vi "ZyklussteuerungGV-11-15.vi"(0 "Traps/MachKoeff0":dbl[](array[numeric]), 1 "DIOsNummern":cluster{"DIOsMod2BNr":i32[]}[](array[cluster]), 3 "FPGA VI Reference In":refnum<k20>, 5 "Traps/MachKoeff1":dbl[](array[numeric]), 7 "ServosWarmHigh (us)KaltHigh(us)":T1, 9 "Traps/MachKoeff2":dbl[](array[numeric]), 11 "Schieberegister":T2, 12 "Zeitpunkte/Setpoints":T4 {"FPGAPID"."proportional gain (Kc)" format="%.11g"; "FPGAPID"."integral gain (Kc*Ts/Ti)" format="%.11g"; "FPGAPID"."derivative gain (Kc*Td/Ts)" format="%.11g"}, 14 "MachKoeffs":T3) -> (4 "Schieberegister":T2)   [LabVIEW 2010]
uses:
  <vilib>/rvi/errors/niLvFpgaWhatHappensToTopLevelVI.ctl
  <vilib>/rvi/interface/common/niFpgaNodeNameForErrorReporting.ctl
  <vilib>/rvi/errors/niLvFpgaAdjustHostInterfaceError.vi
  <vilib>/rvi/interface/nirviReadWriteControl/nirviReadWriteControl.xnode
  GVZwangs.vi
  GVHorstSP.vi
  GVHeizenLH.vi
  GVVentilposition.vi
  GVZeitenZyklen.vi
  C:/Users/HAGAR-IV/Desktop/Zeugs/Johnny/pertrasgc fpga/FPGA-Programm-11-15.vi
  GVZwangsMPV.vi
  GVZwangsMPVPos.vi
  C:/Users/HAGAR-IV/Desktop/Zeugs/markus/version feb 2012/FPGA Bitfiles/pertrasgcfpga2_FPGATarget_FPGA-Programm-11_875D3646.lvbitx
  NiFpgaLv.dll
  <vilib>/Utility/error.llb/Error Cluster From Error Code.vi
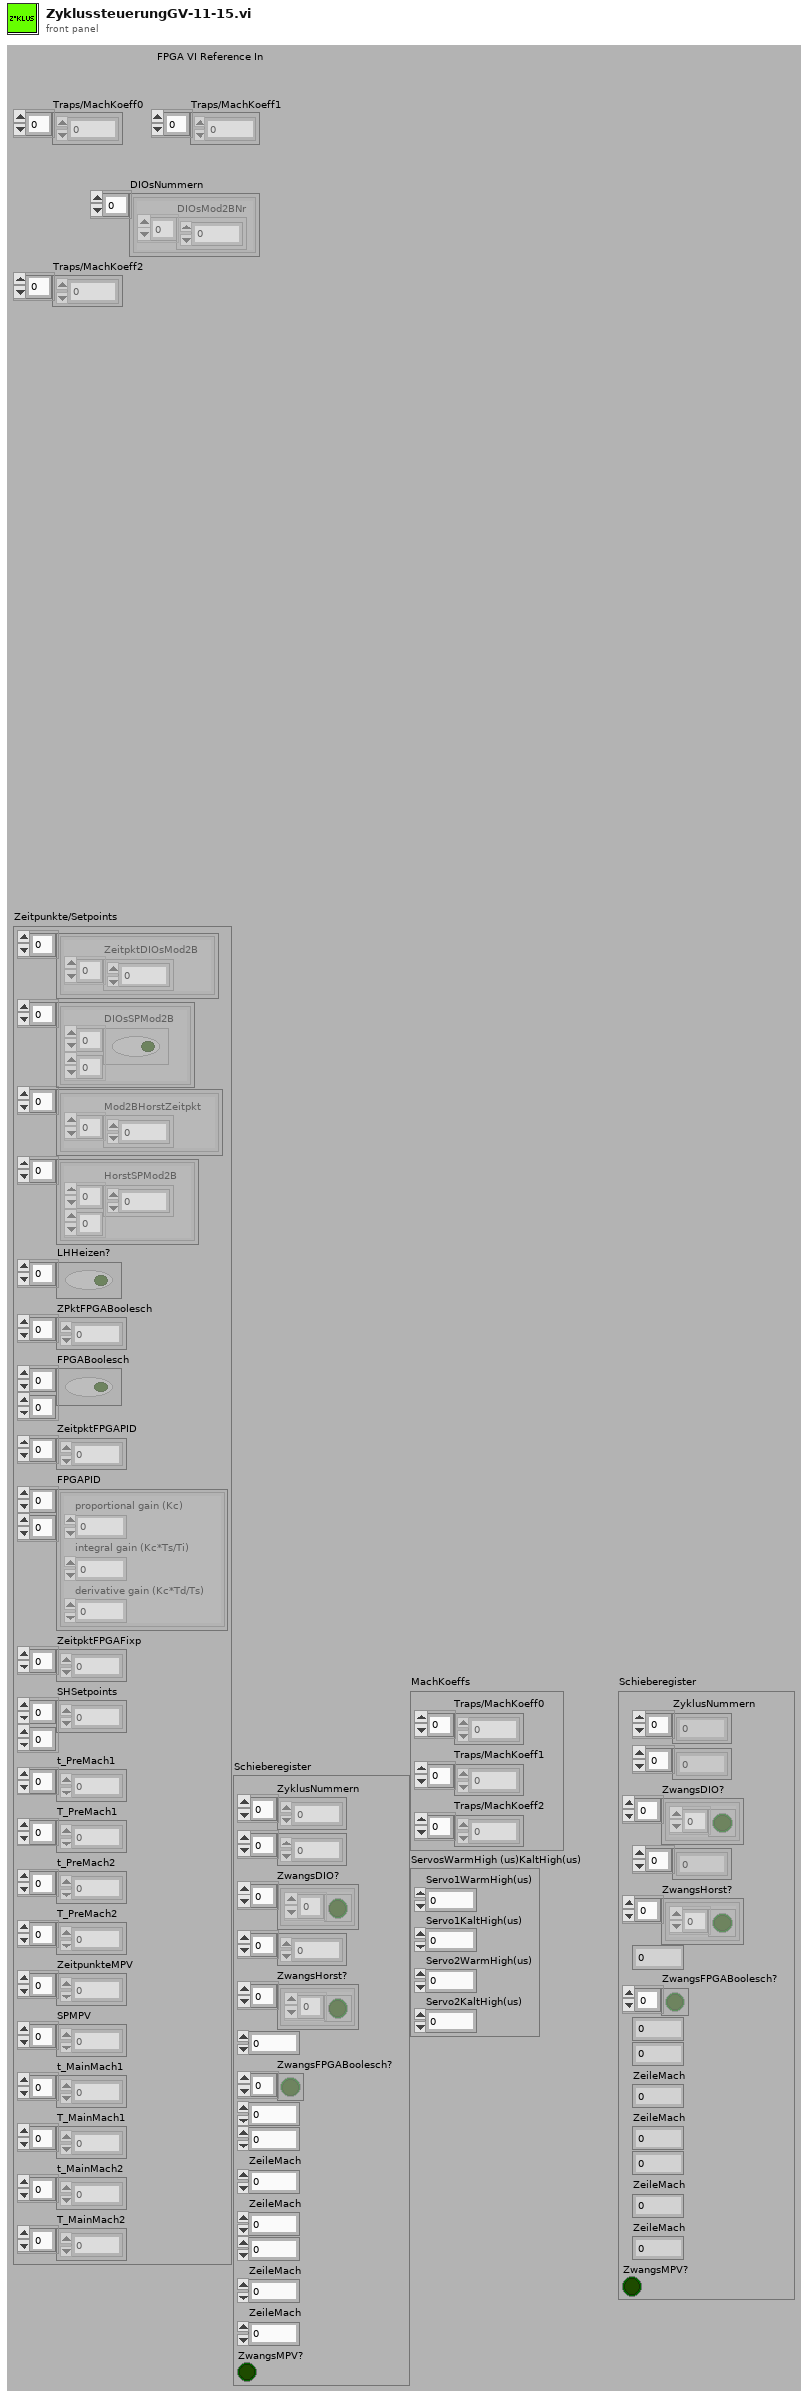
[diagram p1: front panel]
types:
  T1 = cluster{"Servo1WarmHigh(us)":u32, "Servo1KaltHigh(us)":u32, "Servo2WarmHigh(us)":u32, "Servo2KaltHigh(us)":u32}
  T2 = cluster{"ZyklusNummern":i32[], i32[], "ZwangsDIO?":cluster{bool[]}[], i32[], "ZwangsHorst?":cluster{bool[]}[], i32, "ZwangsFPGABoolesch?":bool[], i32, i32, "ZeileMach":i32, "ZeileMach":i32, i32, "ZeileMach":i32, "ZeileMach":i32, "ZwangsMPV?":bool}
  T3 = cluster{"Traps/MachKoeff0":dbl[], "Traps/MachKoeff1":dbl[], "Traps/MachKoeff2":dbl[]}
  T4 = cluster{cluster{"ZeitpktDIOsMod2B":dbl[]}[], cluster{"DIOsSPMod2B":bool[][]}[], cluster{"Mod2BHorstZeitpkt":dbl[]}[], cluster{"HorstSPMod2B":dbl[][]}[], "LHHeizen?":bool[], "ZPktFPGABoolesch":dbl[], "FPGABoolesch":bool[][], "ZeitpktFPGAPID":dbl[], "FPGAPID":cluster{"proportional gain (Kc)":fxp<+/-,16,8>, "integral gain (Kc*Ts/Ti)":fxp<+/-,16,8>, "derivative gain (Kc*Td/Ts)":fxp<+/-,16,8>}[][], "ZeitpktFPGAFixp":dbl[], "SHSetpoints":dbl[][], "t_PreMach1":dbl[], "T_PreMach1":dbl[], "t_PreMach2":dbl[], "T_PreMach2":dbl[], "ZeitpunkteMPV":dbl[], "SPMPV":i32[], "t_MainMach1":dbl[], "T_MainMach1":dbl[], "t_MainMach2":dbl[], "T_MainMach2":dbl[]}
  T5 = cluster{"proportional gain (Kc)":fxp<+/-,16,8>, "integral gain (Kc*Ts/Ti)":fxp<+/-,16,8>, "derivative gain (Kc*Td/Ts)":fxp<+/-,16,8>}[][]
  T6 = cluster{"SpannungenSH[V][0]":fxp<+/-,16,4>, "SpannungenSH[V][1]":fxp<+/-,16,4>, "SpannungenSH[V][2]":fxp<+/-,16,4>, "SpannungenSH[V][3]":fxp<+/-,16,4>}
  T7 = typedef "niFpgaNodeNameForErrorReporting.ctl" = enum16{"Open FPGA VI Reference", "Read/Write Control", "Invoke Method: Abort", "Invoke Method: Acknowledge IRQ", "Invoke Method: Download", "Invoke Method: FIFO.Configure", "Invoke Method: FIFO.Read", "Invoke Method: FIFO.Start", "Invoke Method: FIFO.Stop", "Invoke Method: FIFO.Write", "Invoke Method: Reset", "Invoke Method: Run", "Invoke Method: Wait on IRQ", "Close FPGA VI Reference"}
  T8 = typedef "niLvFpgaWhatHappensToTopLevelVI.ctl" = enum16{"top level VI scripted behind XNode", "top level VI inlined behind XNode"}
  T9 = cluster{"proportional gain (Kc)":fxp<+/-,16,8>, "integral gain (Kc*Ts/Ti)":fxp<+/-,16,8>, "derivative gain (Kc*Td/Ts)":fxp<+/-,16,8>}[]
  T10 = cluster{"FPGAPID[0]":cluster{"proportional gain (Kc)":fxp<+/-,16,8>, "integral gain (Kc*Ts/Ti)":fxp<+/-,16,8>, "derivative gain (Kc*Td/Ts)":fxp<+/-,16,8>}, "FPGAPID[1]":cluster{"proportional gain (Kc)":fxp<+/-,16,8>, "integral gain (Kc*Ts/Ti)":fxp<+/-,16,8>, "derivative gain (Kc*Td/Ts)":fxp<+/-,16,8>}, "FPGAPID[2]":cluster{"proportional gain (Kc)":fxp<+/-,16,8>, "integral gain (Kc*Ts/Ti)":fxp<+/-,16,8>, "derivative gain (Kc*Td/Ts)":fxp<+/-,16,8>}, "FPGAPID[3]":cluster{"proportional gain (Kc)":fxp<+/-,16,8>, "integral gain (Kc*Ts/Ti)":fxp<+/-,16,8>, "derivative gain (Kc*Td/Ts)":fxp<+/-,16,8>}, "FPGAPID[4]":cluster{"proportional gain (Kc)":fxp<+/-,16,8>, "integral gain (Kc*Ts/Ti)":fxp<+/-,16,8>, "derivative gain (Kc*Td/Ts)":fxp<+/-,16,8>}, "FPGAPID[5]":cluster{"proportional gain (Kc)":fxp<+/-,16,8>, "integral gain (Kc*Ts/Ti)":fxp<+/-,16,8>, "derivative gain (Kc*Td/Ts)":fxp<+/-,16,8>}}
  T11 = cluster{"proportional gain (Kc)":fxp<+/-,16,8>, "integral gain (Kc*Ts/Ti)":fxp<+/-,16,8>, "derivative gain (Kc*Td/Ts)":fxp<+/-,16,8>}
  T12 = cluster{"[0]":bool, "[1]":bool, "[2]":bool, "[3]":bool, "[4]":bool, "[5]":bool, "[6]":bool, "[7]":bool, "[8]":bool, "[9]":bool}
  T13 = cluster{"SpannungenSH[V][0]":fxp<+/-,16,4>, "SpannungenSH[V][1]":fxp<+/-,16,4>, "SpannungenSH[V][2]":fxp<+/-,16,4>, "SpannungenSH[V][3]":fxp<+/-,16,4>, "SpannungenSH[V][4]":fxp<+/-,16,4>, "SpannungenSH[V][5]":fxp<+/-,16,4>, "SpannungenSH[V][6]":fxp<+/-,16,4>, "SpannungenSH[V][7]":fxp<+/-,16,4>}
  T14 = cluster{"[0]":bool, "[1]":bool, "[2]":bool, "[3]":bool, "[4]":bool, "[5]":bool, "[6]":bool, "[7]":bool, "[8]":bool, "[9]":bool, "[10]":bool, "[11]":bool, "[12]":bool, "[13]":bool, "[14]":bool, "[15]":bool, "[16]":bool, "[17]":bool, "[18]":bool, "[19]":bool, "[20]":bool, "[21]":bool, "[22]":bool, "[23]":bool, "[24]":bool, "[25]":bool, "[26]":bool, "[27]":bool, "[28]":bool, "[29]":bool, "[30]":bool, "[31]":bool}
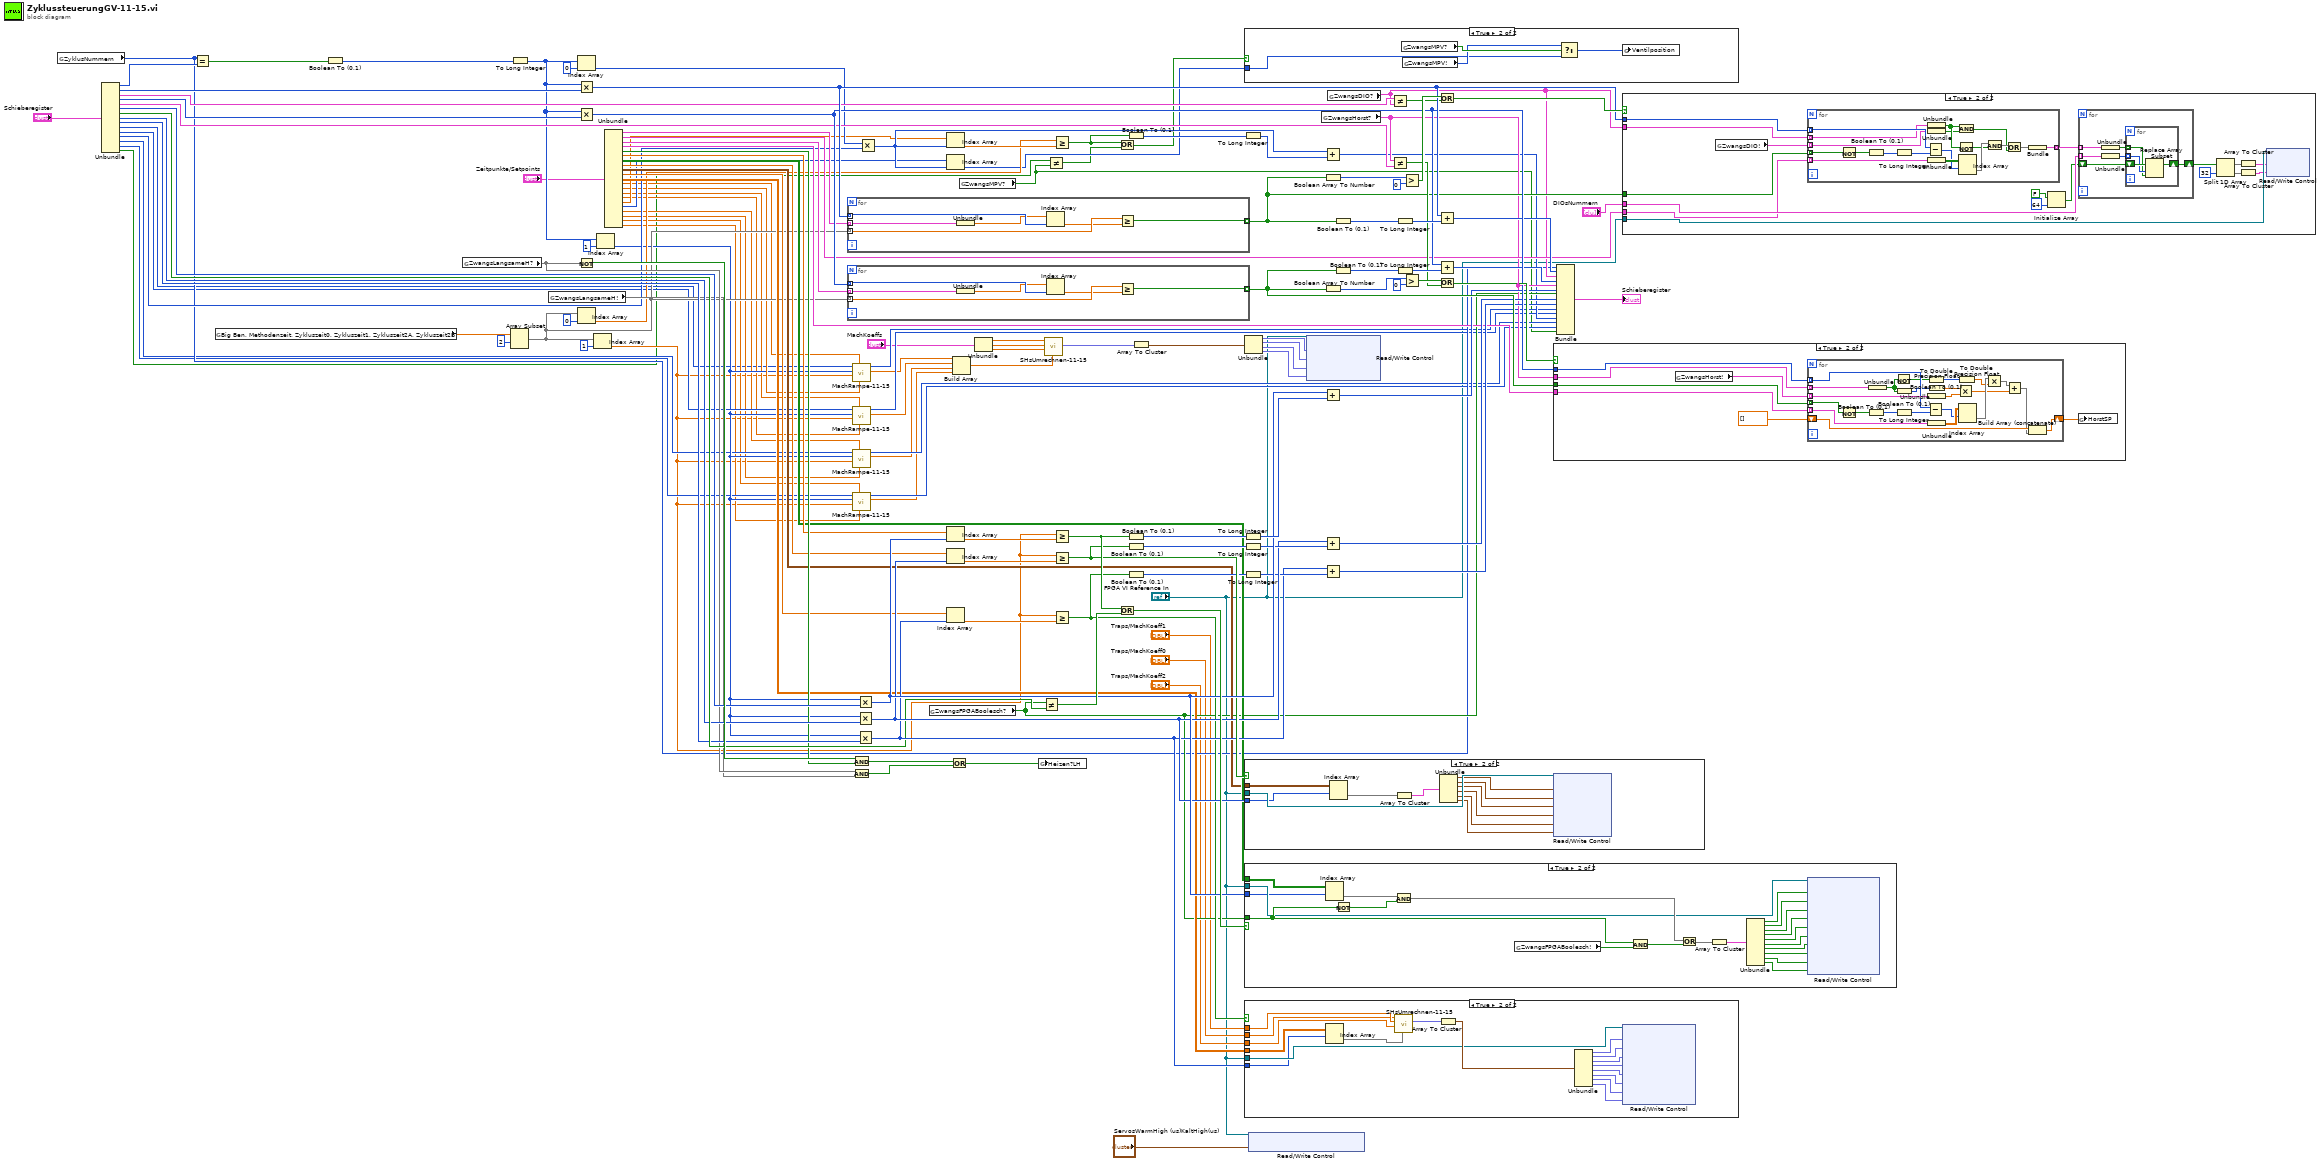
[diagram p0: block diagram]
diagram:
  n1 = global read "GVZeitenZyklen.vi" "ZyklusNummern"() -> (w51:i32[])
  n2 = Unbundle("Schieberegister") -> ("ZyklusNummern"=w95:i32[], w94:i32[], "ZwangsDIO?"=w93:cluster{bool[]}[], w92:i32[], "ZwangsHorst?"=w91:cluster{bool[]}[], w90:i32, "ZwangsFPGABoolesch?"=w89:bool[], w88:i32, w87:i32, "ZeileMach"=w28:i32, "ZeileMach"=w43:i32, w54:i32, "ZeileMach"=w41:i32, "ZeileMach"=w40:i32, "ZwangsMPV?"=w6:bool)
  n3 = Equal?(x=w51, y=w95) -> (x = y?=w138:bool[])
  n4 = global read "GVZeitenZyklen.vi" "Big Ben, Methodenzeit, Zykluszeit0, Zykluszeit1, Zykluszeit2A, Zykluszeit2B"() -> (w49:dbl[])
  n5 = Boolean To (0,1)(Boolean=w138) -> (0, 1=w137:i16[])
  n6 = global read "GVZwangs.vi" "ZwangsLangsameH?"() -> (w68)
  n7 = Array Subset(array=w49, index=2 ("Index")) -> (w48:dbl[])  [unwired: 1 in]
  n8 = To Long Integer(number=w137) -> (32bit integer=w64:i32[])
  n9 = global read "GVZwangs.vi" "ZwangsLangsameH!"() -> (w67)
  n10 = Index Array(array=w64, index=0 ("Index")) -> (element=w62:i32)
  n11 = Index Array(array=w48, index=0 ("Index")) -> (element=w59:dbl)
  n12 = Multiply(x=w64, y=w94) -> (x*y=w103:i32[])
  n13 = Multiply(x=w64, y=w92) -> (x*y=w100:i32[])
  n14 = Not(x=w68) -> (.not. x?=w106:bool)
  n15 = Index Array(array=w48, index=1 ("Index")) -> (element=w29:dbl)
  n16 = Index Array(array=w64, index=1 ("Index")) -> (element=w42:i32)
  n17 = Unbundle("Zeitpunkte/Setpoints") -> (w81:cluster{"ZeitpktDIOsMod2B":dbl[]}[], w80:cluster{"DIOsSPMod2B":bool[][]}[], w79:cluster{"Mod2BHorstZeitpkt":dbl[]}[], w78:cluster{"HorstSPMod2B":dbl[][]}[], "LHHeizen?"=w77:bool[], "ZPktFPGABoolesch"=w76:dbl[], "FPGABoolesch"=w75:bool[][], "ZeitpktFPGAPID"=w74:dbl[], "FPGAPID"=w73:T5, "ZeitpktFPGAFixp"=w72:dbl[], "SHSetpoints"=w71:dbl[][], "t_PreMach1"=w46:dbl[], "T_PreMach1"=w45:dbl[], "t_PreMach2"=w39:dbl[], "T_PreMach2"=w38:dbl[], "ZeitpunkteMPV"=w53:dbl[], "SPMPV"=w52:i32[], "t_MainMach1"=w37:dbl[], "T_MainMach1"=w36:dbl[], "t_MainMach2"=w35:dbl[], "T_MainMach2"=w34:dbl[])
  n18 = for {
    tunnel: w103 -> [w144] mode=indexing
    tunnel: w48 -> [w143] mode=indexing
    tunnel: [w142] -> w97 mode=indexing
    tunnel: w81 -> [w140] mode=indexing
    n19 = Unbundle(w140) -> ("ZeitpktDIOsMod2B"=w139:dbl[])
    n20 = Index Array(array=w139, index=w144) -> (element=w141:dbl)
    n21 = Greater Or Equal?(x=w143, y=w141) -> (x >= y?=w142:bool)
  }
  n22 = for {
    tunnel: w100 -> [w150] mode=indexing
    tunnel: w48 -> [w149] mode=indexing
    tunnel: w79 -> [w146] mode=indexing
    tunnel: [w147] -> w101 mode=indexing
    n23 = Unbundle(w146) -> ("Mod2BHorstZeitpkt"=w145:dbl[])
    n24 = Index Array(array=w145, index=w150) -> (element=w148:dbl)
    n25 = Greater Or Equal?(x=w149, y=w148) -> (x >= y?=w147:bool)
  }
  n26 = call "MachRampe-11-15.vi"("T_Mach"=w45, "t_Mach"=w46, "ZykluszeitMod1"=w29, "gleicherZyklus?"=w42, "ZeileMach"=w28) -> ("T_Mach"=w27:dbl, "ZeileMach"=w44:i32)  [unwired: 5 in]
  n27 = call "MachRampe-11-15.vi"("T_Mach"=w38, "t_Mach"=w39, "ZykluszeitMod1"=w29, "gleicherZyklus?"=w42, "ZeileMach"=w43) -> ("T_Mach"=w26:dbl, "ZeileMach"=w33:i32)  [unwired: 5 in]
  n28 = call "MachRampe-11-15.vi"("T_Mach"=w36, "t_Mach"=w37, "ZykluszeitMod1"=w29, "gleicherZyklus?"=w42, "ZeileMach"=w41) -> ("T_Mach"=w25:dbl, "ZeileMach"=w32:i32)  [unwired: 5 in]
  n29 = call "MachRampe-11-15.vi"("T_Mach"=w34, "t_Mach"=w35, "ZykluszeitMod1"=w29, "gleicherZyklus?"=w42, "ZeileMach"=w40) -> ("T_Mach"=w24:dbl, "ZeileMach"=w31:i32)  [unwired: 5 in]
  n30 = And(x=w106, y=w77) -> (x .and. y?=w105:bool[])
  n31 = And(x=w68, y=w67) -> (x .and. y?=w104:bool)
  n32 = Multiply(x=w42, y=w90) -> (x*y=w117:i32)
  n33 = Multiply(x=w42, y=w88) -> (x*y=w112:i32)
  n34 = Multiply(x=w42, y=w87) -> (x*y=w108:i32)
  n35 = Multiply(x=w62, y=w54) -> (x*y=w56:i32)
  n36 = global read "GVZwangs.vi" "ZwangsFPGABoolesch?"() -> (w65:bool[])
  n37 = Index Array(array=w53, index=w56) -> (element=w60:dbl)
  n38 = Index Array(array=w52, index=w56) -> (element=w9:i32)
  n39 = Index Array(array=w76, index=w117) -> (element=w123:dbl)
  n40 = Index Array(array=w74, index=w112) -> (element=w116:dbl)
  n41 = Index Array(array=w72, index=w108) -> (element=w111:dbl)
  n42 = Or(x=w105, y=w104) -> (x .or. y?=w66:bool[])
  n43 = Build Array(w27, w26, w25, w24) -> (w23:dbl[])
  n44 = global read "GVZwangsMPV.vi" "ZwangsMPV?"() -> (w7:bool)
  n45 = Unbundle("MachKoeffs") -> ("Traps/MachKoeff0"=w18:dbl[], "Traps/MachKoeff1"=w17:dbl[], "Traps/MachKoeff2"=w16:dbl[])
  n46 = global write "GVHeizenLH.vi" "Heizen?LH"(w66) -> ()
  n47 = Not Equal?(x=w65, y=w89) -> (x != y?=w119:bool)
  n48 = call "SHsUmrechnen-11-15.vi"("TemperaturenSH[V]"=w23, "Traps/MachKoeff2"=w16, "Traps/MachKoeff1"=w17, "Traps/MachKoeff0"=w18) -> ("SpannungenSH[V]"=w15:fxp<+/-,16,4>[])  [unwired: 6 in, 1 out]
  n49 = Not Equal?(x=w6, y=w7) -> (x != y?=w5:bool)
  n50 = Greater Or Equal?(x=w59, y=w60) -> (x >= y?=w4:bool)
  n51 = Greater Or Equal?(x=w29, y=w123) -> (x >= y?=w120:bool)
  n52 = Greater Or Equal?(x=w29, y=w116) -> (x >= y?=w113:bool)
  n53 = Greater Or Equal?(x=w29, y=w111) -> (x >= y?=w107:bool)
  n54 = Or(x=w4, y=w5) -> (x .or. y?=w3:bool)
  n55 = Or(x=w120, y=w119) -> (x .or. y?=w118:bool)
  n56 = Boolean To (0,1)(Boolean=w4) -> (0, 1=w58:i16)
  n57 = Boolean To (0,1)(Boolean=w120) -> (0, 1=w122:i16)
  n58 = Boolean To (0,1)(Boolean=w113) -> (0, 1=w115:i16)
  n59 = Boolean To (0,1)(Boolean=w107) -> (0, 1=w110:i16)
  n60 = Array To Cluster(array=w15) -> (cluster=w14:T6)
  n61 = To Long Integer(number=w58) -> (32bit integer=w57:i32)
  n62 = To Long Integer(number=w122) -> (32bit integer=w121:i32)
  n63 = To Long Integer(number=w115) -> (32bit integer=w114:i32)
  n64 = To Long Integer(number=w110) -> (32bit integer=w109:i32)
  n65 = case shown="True" w3 {
    tunnel: w9 -> [_ w152]
    frame False {
    }
    frame True {
      n66 = global read "GVZwangsMPV.vi" "ZwangsMPV?"() -> (w154:bool)
      n67 = global read "GVZwangsMPVPos.vi" "ZwangsMPV!"() -> (w153:i32)
      n68 = Select(t=w153, s=w154, f=w152) -> (s? t:f=w151:i32)
      n69 = global write "GVVentilposition.vi" "Ventilposition"(w151) -> ()
    }
  }
  n70 = Unbundle(w14) -> ("SpannungenSH[V][0]"=w13:fxp<+/-,16,4>, "SpannungenSH[V][1]"=w12:fxp<+/-,16,4>, "SpannungenSH[V][2]"=w11:fxp<+/-,16,4>, "SpannungenSH[V][3]"=w10:fxp<+/-,16,4>)
  n71 = case shown="True" w113 {
    tunnel: "FPGA VI Reference In" -> [_ w165]
    tunnel: w73 -> [_ w164]
    tunnel: w112 -> [_ w157]
    frame False {
    }
    frame True {
      n72 = Index Array(array=w164, index (row)=w157) -> (element=w163:T9)  [unwired: 1 in]
      n73 = Array To Cluster(array=w163) -> (cluster=w162:T10)
      n74 = Unbundle(w162) -> ("FPGAPID[0]"=w161:T11, "FPGAPID[1]"=w160:T11, "FPGAPID[2]"=w159:T11, "FPGAPID[3]"=w158:T11, "FPGAPID[4]"=w156:T11, "FPGAPID[5]"=w155:T11)
      n75 = xnode "Read/Write Control"("FPGA VI Reference In"=w165, "PIDTrap1"=w161, "PIDTrap2"=w160, "PIDPreMach1"=w159, "PIDPreMach2"=w158, "PIDMainMach1"=w156, "PIDMainMach2"=w155) -> ()  [unwired: 1 in, 2 out]
    }
  }
  n76 = case shown="True" w118 {
    tunnel: w117 -> [_ w350]
    tunnel: w65 -> [_ w355]
    tunnel: w75 -> [_ w359]
    tunnel: "FPGA VI Reference In" -> [_ w352]
    frame False {
    }
    frame True {
      n77 = Index Array(array=w359, index (row)=w350) -> (element=w357:bool[])  [unwired: 1 in]
      n78 = Not(x=w355) -> (.not. x?=w358:bool[])
      n79 = And(x=w357, y=w358) -> (x .and. y?=w356:bool[])
      n80 = global read "GVZwangs.vi" "ZwangsFPGABoolesch!"() -> (w349:bool[])
      n81 = And(x=w355, y=w349) -> (x .and. y?=w354:bool[])
      n82 = Or(x=w356, y=w354) -> (x .or. y?=w353:bool[])
      n83 = Array To Cluster(array=w353) -> (cluster=w351:T12)
      n84 = Unbundle(w351) -> ("[0]"=w348:bool, "[1]"=w347:bool, "[2]"=w346:bool, "[3]"=w345:bool, "[4]"=w344:bool, "[5]"=w343:bool, "[6]"=w342:bool, "[7]"=w341:bool, "[8]"=w340:bool, "[9]"=w339:bool)
      n85 = xnode "Read/Write Control"("FPGA VI Reference In"=w352, "Servo1An?"=w348, "Servo2An?"=w347, "ServoTrap1kalt"=w346, "ServoTrap2kalt"=w345, "Heizen?Trap1"=w344, "Heizen?Trap2"=w343, "Heizen?PreMach1"=w342, "Heizen?PreMach2"=w341, "Heizen?MainMach1"=w340, "Heizen?MainMach2"=w339) -> ()  [unwired: 1 in, 2 out]
    }
  }
  n86 = case shown="True" w107 {
    tunnel: w108 -> [_ w600]
    tunnel: w71 -> [_ w603]
    tunnel: "FPGA VI Reference In" -> [_ w601]
    tunnel: "Traps/MachKoeff2" -> [_ w589]
    tunnel: "Traps/MachKoeff1" -> [_ w588]
    tunnel: "Traps/MachKoeff0" -> [_ w587]
    frame False {
    }
    frame True {
      n87 = Index Array(array=w603, index (row)=w600) -> (element=w594:dbl[])  [unwired: 1 in]
      n88 = call "SHsUmrechnen-11-15.vi"("TemperaturenSH[V]"=w594, "Traps/MachKoeff2"=w589, "Traps/MachKoeff1"=w588, "Traps/MachKoeff0"=w587) -> ("SpannungenSH[V]"=w595:fxp<+/-,16,4>[])  [unwired: 6 in, 1 out]
      n89 = Array To Cluster(array=w595) -> (cluster=w602:T13)
      n90 = Unbundle(w602) -> ("SpannungenSH[V][0]"=w599:fxp<+/-,16,4>, "SpannungenSH[V][1]"=w598:fxp<+/-,16,4>, "SpannungenSH[V][2]"=w597:fxp<+/-,16,4>, "SpannungenSH[V][3]"=w596:fxp<+/-,16,4>, "SpannungenSH[V][4]"=w593:fxp<+/-,16,4>, "SpannungenSH[V][5]"=w592:fxp<+/-,16,4>, "SpannungenSH[V][6]"=w591:fxp<+/-,16,4>, "SpannungenSH[V][7]"=w590:fxp<+/-,16,4>)
      n91 = xnode "Read/Write Control"("FPGA VI Reference In"=w601, "UTempSPTrap1"=w599, "UTempMaxTrap1"=w598, "UTempSPTrap2"=w597, "UTempMaxTrap2"=w596, "Umax[V]PreMach1"=w593, "Umax[V]PreMach2"=w592, "Umax[V]MainMach1"=w591, "Umax[V]MainMach2"=w590) -> ()  [unwired: 1 in, 2 out]
    }
  }
  n92 = xnode "Read/Write Control"("FPGA VI Reference In"="FPGA VI Reference In", "ServosWarmHigh (us)KaltHigh(us)"="ServosWarmHigh (us)KaltHigh(us)") -> ()  [unwired: 1 in, 2 out]
  n93 = xnode "Read/Write Control"("FPGA VI Reference In"="FPGA VI Reference In", "USetp[V]PreMach1"=w13, "USetp[V]PreMach2"=w12, "USetp[V]MainMach1"=w11, "USetp[V]MainMach2"=w10) -> ()  [unwired: 1 in, 2 out]
  n94 = global read "GVZwangs.vi" "ZwangsHorst?"() -> (w69:cluster{bool[]}[])
  n95 = Add(x=w56, y=w57) -> (x+y=w55:i32)
  n96 = Add(x=w117, y=w121) -> (x+y=w84:i32)
  n97 = Add(x=w112, y=w114) -> (x+y=w83:i32)
  n98 = Add(x=w108, y=w109) -> (x+y=w82:i32)
  n99 = Boolean Array To Number(Boolean array=w97) -> (number=w134:u32)
  n100 = Boolean Array To Number(Boolean array=w101) -> (number=w128:u32)
  n101 = global read "GVZwangs.vi" "ZwangsDIO?"() -> (w70:cluster{bool[]}[])
  n102 = Boolean To (0,1)(Boolean=w97) -> (0, 1=w136:i16[])
  n103 = Boolean To (0,1)(Boolean=w101) -> (0, 1=w130:i16[])
  n104 = Not Equal?(x=w93, y=w70) -> (x != y?=w98:bool)
  n105 = Not Equal?(x=w69, y=w91) -> (x != y?=w99:bool)
  n106 = To Long Integer(number=w136) -> (32bit integer=w135:i32[])
  n107 = To Long Integer(number=w130) -> (32bit integer=w129:i32[])
  n108 = Greater?(x=w134, y=u32 0) -> (0:w131:bool)
  n109 = Greater?(x=w128, y=u32 0) -> (0:w126:bool)
  n110 = Or(x=w131, y=w98) -> (x .or. y?=w132:bool)
  n111 = Add(x=w103, y=w135) -> (x+y=w86:i32[])
  n112 = Add(x=w100, y=w129) -> (x+y=w85:i32[])
  n113 = Or(x=w126, y=w99) -> (x .or. y?=w102:bool)
  n114 = case shown="True" w102 {
    tunnel: w78 -> [_ w848]
    tunnel: w69 -> [_ w849]
    tunnel: w101 -> [_ w851]
    tunnel: w100 -> [_ w850]
    frame False {
    }
    frame True {
      n115 = global read "GVZwangs.vi" "ZwangsHorst!"() -> (w846:cluster{dbl[]}[])
      n116 = for {
        tunnel: w851 -> [w871] mode=indexing
        tunnel: w850 -> [w868] mode=indexing
        tunnel: w849 -> [w874] mode=indexing
        tunnel: w848 -> [w872] mode=indexing
        tunnel: w846 -> [w873] mode=indexing
        shift-right: [w852] -> w845
        shift-left: dbl[] [] -> [w854]
        n117 = Not(x=w871) -> (.not. x?=w870:bool)
        n118 = Boolean To (0,1)(Boolean=w870) -> (0, 1=w869:i16)
        n119 = Unbundle(w874) -> (w861:bool[])
        n120 = Not(x=w861) -> (.not. x?=w864:bool[])
        n121 = Boolean To (0,1)(Boolean=w861) -> (0, 1=w862:i16[])
        n122 = To Long Integer(number=w869) -> (32bit integer=w867:i32)
        n123 = Subtract(x=w868, y=w867) -> (x-y=w865:i32)
        n124 = Boolean To (0,1)(Boolean=w864) -> (0, 1=w863:i16[])
        n125 = To Double Precision Float(number=w862) -> (double precision float=w858:dbl[])
        n126 = Unbundle(w873) -> (w857:dbl[])
        n127 = Unbundle(w872) -> ("HorstSPMod2B"=w866:dbl[][])
        n128 = Multiply(x=w858, y=w857) -> (x*y=w855:dbl[])
        n129 = To Double Precision Float(number=w863) -> (double precision float=w859:dbl[])
        n130 = Index Array(array=w866, index (row)=w865) -> (element=w860:dbl[])  [unwired: 1 in]
        n131 = Multiply(x=w860, y=w859) -> (x*y=w856:dbl[])
        n132 = Add(x=w856, y=w855) -> (x+y=w853:dbl[])
        n133 = Build Array (concatenate)(w854, w853) -> (w852:dbl[])
      }
      n134 = global write "GVHorstSP.vi" "HorstSP"(w845) -> ()
    }
  }
  n135 = Bundle("ZyklusNummern"=w51, w86, "ZwangsDIO?"=w70, w85, "ZwangsHorst?"=w69, w84, "ZwangsFPGABoolesch?"=w65, w83, w82, "ZeileMach"=w44, "ZeileMach"=w33, w55, "ZeileMach"=w32, "ZeileMach"=w31, "ZwangsMPV?"=w7) -> (→"Schieberegister":T2)  [unwired: 1 in]
  n136 = case shown="True" w132 {
    tunnel: w103 -> [_ w887]
    tunnel: w70 -> [_ w884]
    tunnel: "DIOsNummern" -> [_ w891]
    tunnel: "FPGA VI Reference In" -> [_ w890]
    tunnel: w80 -> [_ w885]
    tunnel: w97 -> [_ w886]
    frame False {
    }
    frame True {
      n137 = global read "GVZwangs.vi" "ZwangsDIO!"() -> (w875:cluster{bool[]}[])
      n138 = for {
        tunnel: w887 -> [w906] mode=indexing
        tunnel: w886 -> [w905] mode=indexing
        tunnel: w885 -> [w904] mode=indexing
        tunnel: w884 -> [w903] mode=indexing
        tunnel: w875 -> [w902] mode=indexing
        tunnel: [w892] -> w883 mode=indexing
        n139 = Not(x=w905) -> (.not. x?=w908:bool)
        n140 = Boolean To (0,1)(Boolean=w908) -> (0, 1=w907:i16)
        n141 = To Long Integer(number=w907) -> (32bit integer=w909:i32)
        n142 = Subtract(x=w906, y=w909) -> (x-y=w900:i32)
        n143 = Unbundle(w903) -> (w897:bool[])
        n144 = Unbundle(w902) -> (w896:bool[])
        n145 = Unbundle(w904) -> ("DIOsSPMod2B"=w901:bool[][])
        n146 = And(x=w897, y=w896) -> (x .and. y?=w894:bool[])
        n147 = Not(x=w897) -> (.not. x?=w898:bool[])
        n148 = Index Array(array=w901, index (row)=w900) -> (element=w899:bool[])  [unwired: 1 in]
        n149 = And(x=w899, y=w898) -> (x .and. y?=w895:bool[])
        n150 = Or(x=w895, y=w894) -> (x .or. y?=w893:bool[])
        n151 = Bundle(w893) -> (w892:cluster{bool[]})  [unwired: 1 in]
      }
      n152 = Initialize Array(FALSE, 64 ("Dimension")) -> (w876:bool[])
      n153 = for {
        tunnel: w883 -> [w984] mode=indexing
        tunnel: w891 -> [w986] mode=indexing
        shift-right: [w987] -> w888
        shift-left: w876 -> [w988]
        n154 = Unbundle(w984) -> (w983:bool[])
        n155 = Unbundle(w986) -> ("DIOsMod2BNr"=w985:i32[])
        n156 = for {
          tunnel: w983 -> [w990] mode=indexing
          tunnel: w985 -> [w991] mode=indexing
          shift-right: [w989] -> w987
          shift-left: w988 -> [w992]
          n157 = Replace Array Subset(array=w992, new element=w990, index=w991) -> (w989:bool[])
        }
      }
      n158 = Split 1D Array(array=w888, index=32 ("Länge")) -> (first subarray=w882:bool[], second subarray=w880:bool[])
      n159 = Array To Cluster(array=w882) -> (cluster=w881:T14)
      n160 = Array To Cluster(array=w880) -> (cluster=w879:T14)
      n161 = xnode "Read/Write Control"("FPGA VI Reference In"=w890, "Mod5/DIO"=w881, "Mod6/DIO"=w879) -> ()  [unwired: 1 in, 2 out]
    }
  }
